vi "CPP-6068Special.vi"() -> (5 "Plug in titles":string[](array[string]), 7 "Plug in values":string[](array[string]))   [LabVIEW 2011]
uses:
  Globals/Meas_global.vi
  CPP/ProjectSpecific/6068-VeerTowers/MesowestParse/MetDataGlobal.vi
  Globals/Constants_global.vi
panel:
  out "Results":string[][](table)
  in  "OutputFile":path
  out "BlockStartTime":dbl format="%#_12f"
  in  "SearchBands":cluster{"Min":dbl, "Max":dbl, "Name":string}[](array[cluster])=[{"Min"=40.0, "Max"=70.0, "Name"="60Hz:Band"}, {"Min"=100.0, "Max"=140.0, "Name"="120Hz:Band"}, {"Min"=450.0, "Max"=510.0, "Name"="480Hz:Band"}, {"Min"=600.0, "Max"=680.0, "Name"="640Hz:Band"}, {"Min"=520.0, "Max"=590.0, "Name"="550Hz:Band"}]
  out "TimeRunStarted":dbl format="%^<%H:%M:%S\n%x %Z>T"
  out "Processing last block?":bool
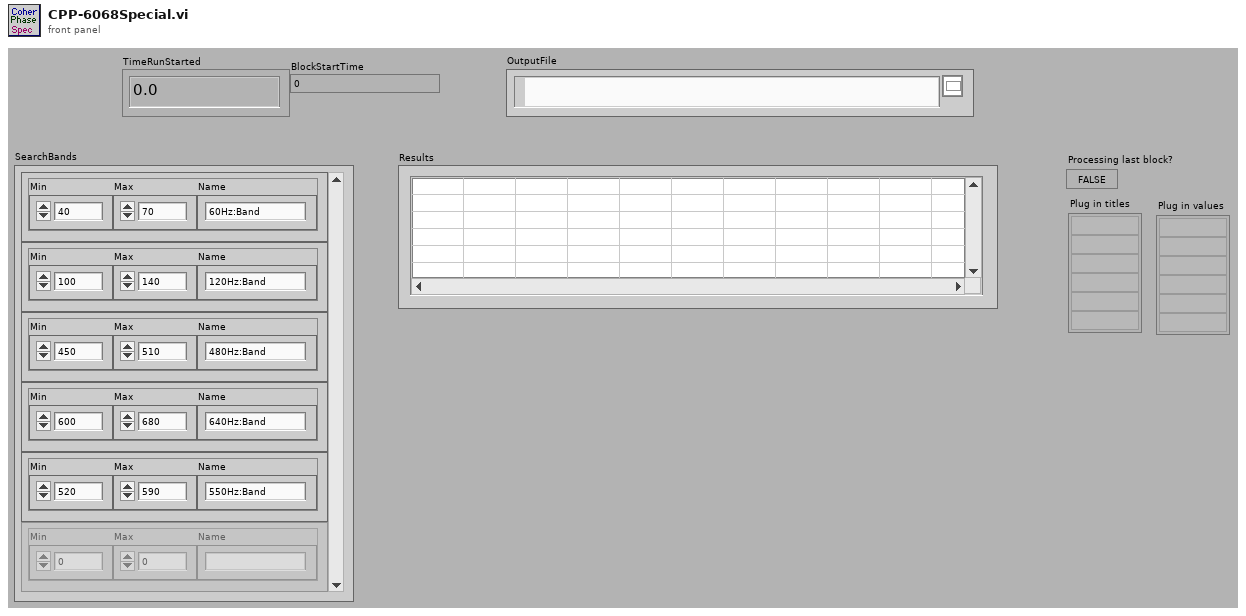
[diagram p1: front panel]
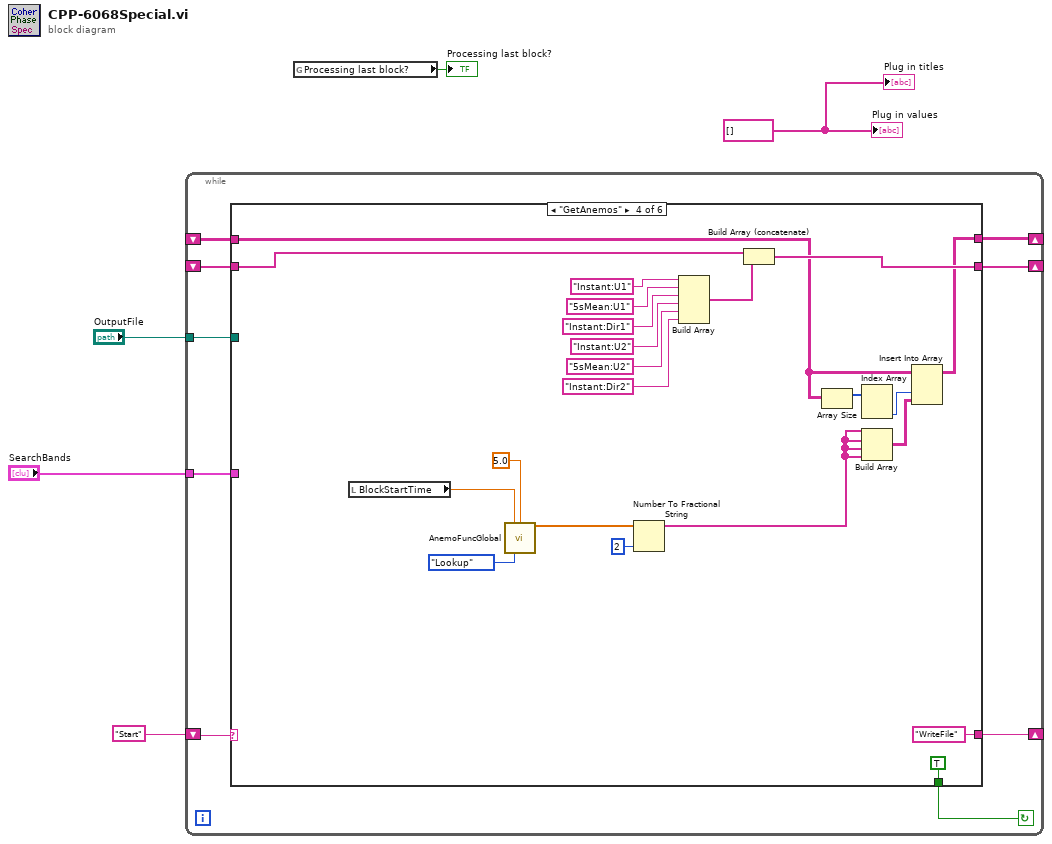
[diagram p0: block diagram]
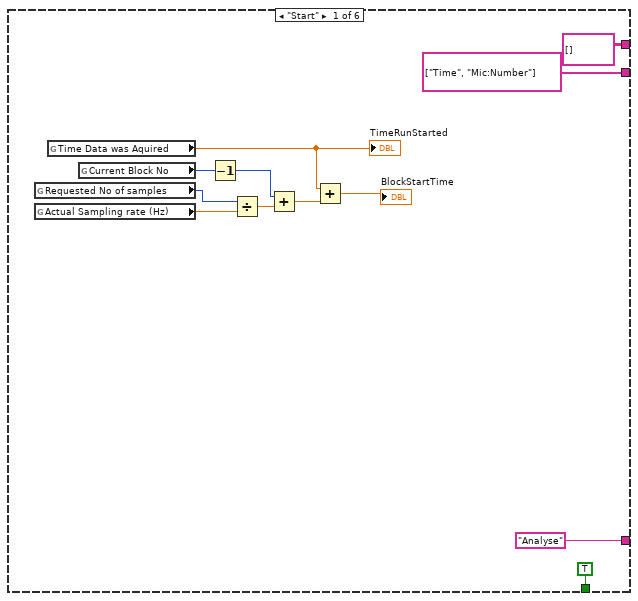
[diagram p2: hidden frame]
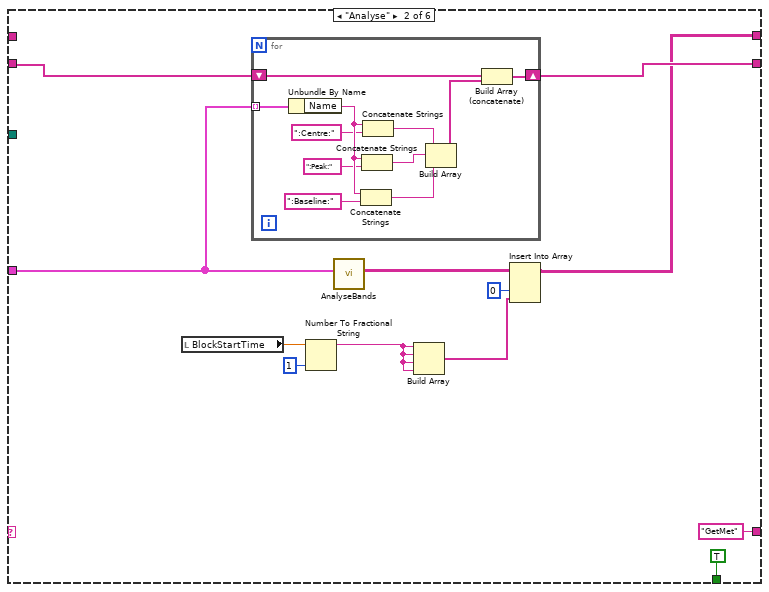
[diagram p3: hidden frame]
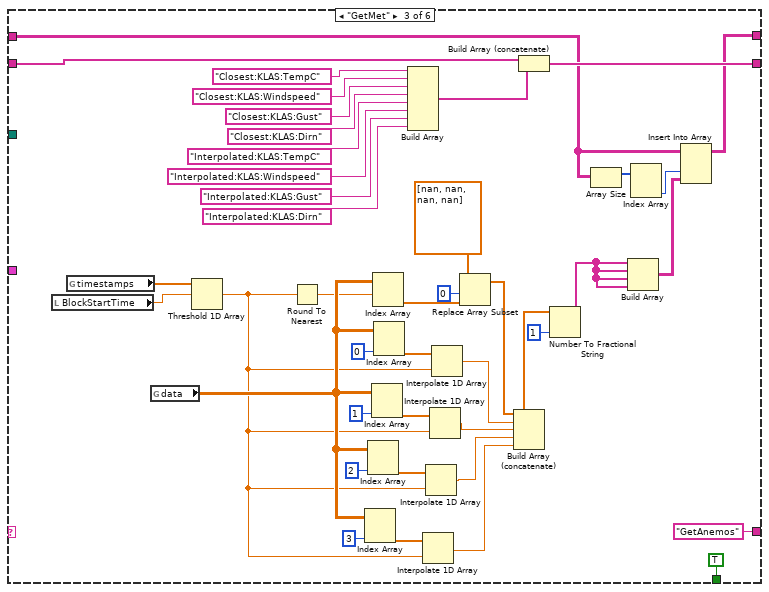
[diagram p4: hidden frame]
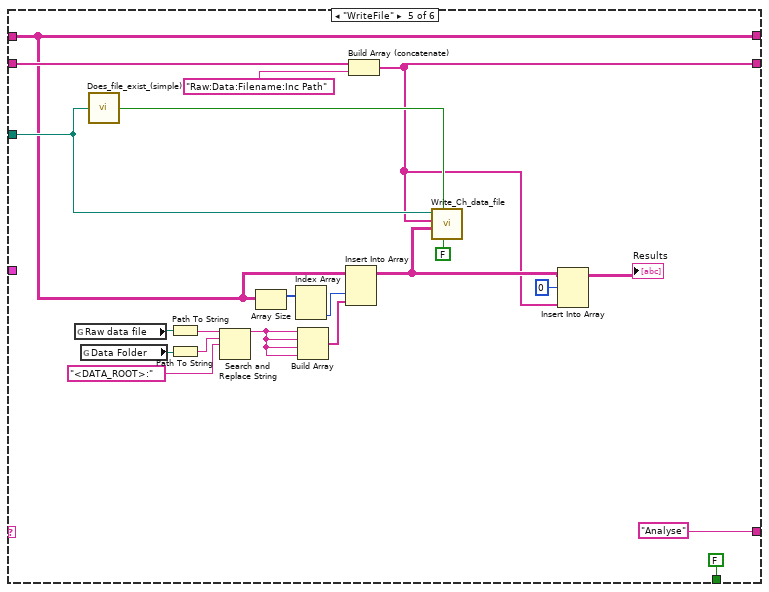
[diagram p5: hidden frame]
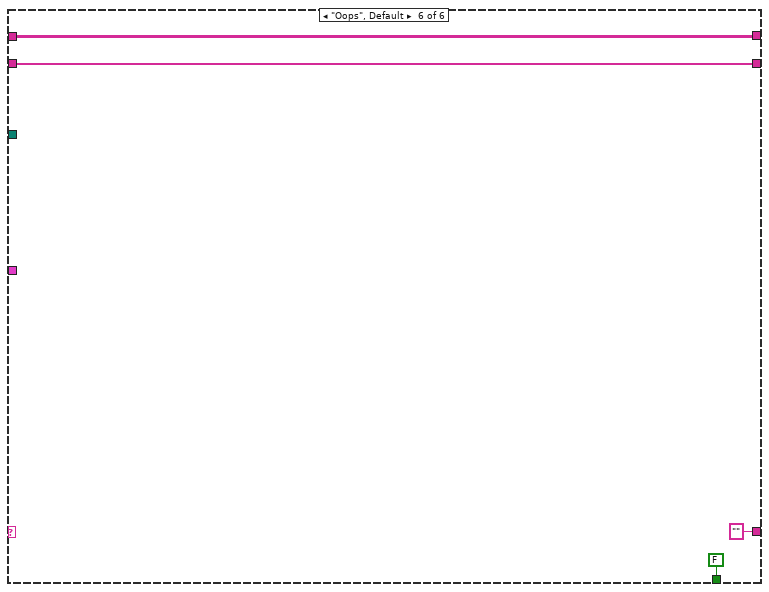
[diagram p6: hidden frame]
diagram:
  w4 = string[] [] ("Add in values")
  n1 = while {
    tunnel: "SearchBands" -> [w14]
    shift-right: [w12] -> _
    shift-left: "Start" -> [w13]
    shift-right: [w9] -> _
    shift-left: _ -> [w10]
    shift-right: [w7] -> _
    shift-left: _ -> [w8]
    tunnel: "OutputFile" -> [w6]
    stop <- w11 continue-if-true
    n2 = case shown="\"GetAnemos\"" w13 {
      tunnel: w14 -> [_ w32 _ _ _ _]
      tunnel: ["Analyse" "GetMet" "GetAnemos" "WriteFile" "Analyse" ""] -> w12
      tunnel: [TRUE TRUE TRUE TRUE FALSE FALSE] -> w11
      tunnel: w10 -> [_ w31 w63 w104 w119 w136]
      tunnel: [string[] ["Time", "Mic:Number"] w30 w62 w103 w117 w136] -> w9
      tunnel: [string[][] [] ("Results") w29 w57 w100 w114 w135] -> w7
      tunnel: w8 -> [_ _ w59 w99 w114 w135]
      tunnel: w6 -> [_ _ _ _ w121 _]
      frame "Start" {
        n3 = global read "Meas_global.vi" "Requested No of samples"() -> (w24:i32)
        n4 = global read "Meas_global.vi" "Actual Sampling rate (Hz)"() -> (w23:dbl)
        n5 = global read "Meas_global.vi" "Time Data was Aquired"() -> (w19:dbl)
        "TimeRunStarted" <- w19
        n6 = global read "Meas_global.vi" "Current Block No"() -> (w25:i32)
        n7 = Decrement(x=w25) -> (x-1=w21:i32)
        n8 = Divide(x=w24, y=w23) -> (x/y=w22:dbl)
        n9 = Add(x=w21, y=w22) -> (x+y=w20:dbl)
        n10 = Add(x=w19, y=w20) -> (x+y=→"BlockStartTime":dbl)
      }
      frame "Analyse" {
        n11 = local read "BlockStartTime"() -> (w33:dbl)
        n12 = for {
          shift-right: [w41] -> w30
          shift-left: w31 -> [w39]
          tunnel: w32 -> [w49] mode=indexing
          n13 = Unbundle By Name(w49) -> ("Name"=w48:string)
          n14 = Concatenate Strings(w48, ":Baseline:" ("string")) -> (w42:string)
          n15 = Concatenate Strings(w48, ":Peak:" ("string")) -> (w43:string)
          n16 = Concatenate Strings(w48, ":Centre:" ("string")) -> (w44:string)
          n17 = Build Array(w44, w43, w42) -> (w40:string[])
          n18 = Build Array (concatenate)(w39, w40) -> (w41:string[])
        }
        n19 = Number To Fractional String(number=w33, precision (6)=i16 1) -> (F-format string=w28:string)  [unwired: 2 in]
        n20 = call "AnalyseBands.vi"("SearchBands"=w32) -> ("Results"=w38:string[][])  [unwired: 10 in]
        n21 = Build Array(w28, w28, w28, w28) -> (w37:string[])
        n22 = Insert Into Array(array=w38, index (col)=0 ("disabled index (col)"), new element=w37) -> (w29:string[][])  [unwired: 1 in]
      }
      frame "GetMet" {
        n23 = local read "BlockStartTime"() -> (w88:dbl)
        n24 = global read "MetDataGlobal.vi" "timestamps"() -> (w91:dbl[])
        n25 = global read "MetDataGlobal.vi" "data"() -> (w75:dbl[][])
        n26 = Threshold 1D Array(2:w88, 3:w91) -> (0:w74:dbl)  [unwired: 1 in]
        n27 = Round To Nearest(number=w74) -> (nearest integer value=w73:dbl)
        n28 = Index Array(array=w75, index (col)=3 ("disabled index (col)")) -> (element=w81:dbl[])  [unwired: 1 in]
        n29 = Index Array(array=w75, index (col)=2 ("disabled index (col)")) -> (element=w82:dbl[])  [unwired: 1 in]
        n30 = Index Array(array=w75, index (col)=1 ("disabled index (col)")) -> (element=w85:dbl[])  [unwired: 1 in]
        n31 = Index Array(array=w75, index (row)=w73) -> (element=w54:dbl[])  [unwired: 1 in]
        n32 = Index Array(array=w75, index (col)=0 ("disabled index (col)")) -> (element=w86:dbl[])  [unwired: 1 in]
        n33 = Build Array("Closest:KLAS:TempC", "Closest:KLAS:Windspeed", "Closest:KLAS:Gust", "Closest:KLAS:Dirn", "Interpolated:KLAS:TempC", "Interpolated:KLAS:Windspeed", "Interpolated:KLAS:Gust", "Interpolated:KLAS:Dirn") -> (w64:string[])
        n34 = Interpolate 1D Array(1:w74, 2:w81) -> (0:w76:dbl)
        n35 = Interpolate 1D Array(1:w74, 2:w82) -> (0:w77:dbl)
        n36 = Interpolate 1D Array(1:w74, 2:w85) -> (0:w78:dbl)
        n37 = Interpolate 1D Array(1:w74, 2:w86) -> (0:w79:dbl)
        n38 = Replace Array Subset(array=dbl[] [nan, nan, nan, nan], new element=w54, index=0) -> (w55:dbl[])
        n39 = Build Array (concatenate)(w55, w79, w78, w77, w76) -> (w61:dbl[])
        n40 = Build Array (concatenate)(w63, w64) -> (w62:string[])
        n41 = Number To Fractional String(number=w61, precision (6)=i16 1) -> (F-format string=w51:string[])  [unwired: 2 in]
        n42 = Array Size(array=w59) -> (size(s)=w58:i32[])
        n43 = Build Array(w51, w51, w51, w51) -> (w60:string[][])
        n44 = Index Array(array=w58) -> (element #2=w56:i32)  [unwired: 2 in, 1 out]
        n45 = Insert Into Array(array=w59, index (col)=w56, new element=w60) -> (w57:string[][])  [unwired: 1 in]
      }
      frame "GetAnemos" {
        n46 = local read "BlockStartTime"() -> (w98:dbl)
        n47 = call "AnemoFuncGlobal.vi"("searchValue"=w98, "history(samples)"=5.0 ("fractional index or x"), "Mode"=enum16{"Overwrite", "Append", "Read", "Lookup"}."Lookup") -> ("results"=w96:dbl[])  [unwired: 12 in]
        n48 = Number To Fractional String(number=w96, precision (6)=i16 2) -> (F-format string=w93:string[])  [unwired: 2 in]
        n49 = Build Array("Instant:U1", "5sMean:U1", "Instant:Dir1", "Instant:U2", "5sMean:U2", "Instant:Dir2") -> (w105:string[])
        n50 = Build Array (concatenate)(w104, w105) -> (w103:string[])
        n51 = Array Size(array=w99) -> (size(s)=w102:i32[])
        n52 = Index Array(array=w102) -> (element #2=w101:i32)  [unwired: 2 in, 1 out]
        n53 = Build Array(w93, w93, w93, w93) -> (w94:string[][])
        n54 = Insert Into Array(array=w99, index (col)=w101, new element=w94) -> (w100:string[][])  [unwired: 1 in]
      }
      frame "WriteFile" {
        n55 = global read "Meas_global.vi" "Raw data file"() -> (w127:path)
        n56 = global read "Constants_global.vi" "Data Folder"() -> (w126:path)
        n57 = call "Does_file_exist_(simple).vi"("Pathname"=w121) -> ("exists?"=w132:bool)
        n58 = Path To String(path=w127) -> (string=w125:string)
        n59 = Path To String(path=w126) -> (string=w124:string)
        n60 = Search and Replace String(input string=w125, search string=w124, replace string="<DATA_ROOT>:" ("replace string (\"\")")) -> (result string=w123:string)  [unwired: 5 in, 3 out]
        n61 = Array Size(array=w114) -> (size(s)=w129:i32[])
        n62 = Index Array(array=w129) -> (element #2=w128:i32)  [unwired: 2 in, 1 out]
        n63 = Build Array(w123, w123, w123, w123) -> (w130:string[])
        n64 = Insert Into Array(array=w114, index (col)=w128, new element=w130) -> (w118:string[][])  [unwired: 1 in]
        n65 = Build Array (concatenate)(w119, "Raw:Data:Filename:Inc Path") -> (w117:string[])
        n66 = call "Write_Ch_data_file.vi"("Lock File"=FALSE, "exists?"=w132, "Channel Values"=w118, "Channel names"=w117, "Filename"=w121) -> ()  [unwired: 7 in]
        n67 = Insert Into Array(array=w118, index (row)=0, new element=w117) -> (→"Results":string[][])  [unwired: 1 in]
      }
      frame "Oops", Default {
      }
    }
  }
  n68 = global read "Meas_global.vi" "Processing last block?"() -> (→"Processing last block?":bool)
  "Plug in titles" <- w4
  "Plug in values" <- w4
